vi "Decay Fitter.vi"() -> ()   [LabVIEW 2014]
uses:
  <vilib>/Utility/file.llb/Read From Spreadsheet File (DBL).vi
panel:
  out "time constant":dbl=122.42486013356687
  in  "file path (dialog if empty)":path=path "C:/Users/zchmlk/Desktop/week8-master/Decay2.txt"
  out "Decay Rate Fit":cluster{"all rows":dbl[], "all rows":dbl[]}[](graph)=[{"all rows"=[0.0, 1.0, 2.0, 3.0, 4.0, 5.0, 6.0, 7.0, 8.0, 9.0, 10.0, 11.0, 12.0, 13.0, 14.0, 15.0, 16.0, 17.0, 18.0, 19.0, 20.0, 21.0, 22.0, 23.0, 24.0, 25.0, 26.0, 27.0, 28.0, 29.0, 30.0, 31.0, 32.0, 33.0, 34.0, 35.0, 36.0, 37.0, 38.0, 39.0, 40.0, 41.0, 42.0, 43.0, 44.0, 45.0, 46.0, 47.0, 48.0, 49.0, 50.0, 51.0, 52.0, 53.0, 54.0, 55.0, 56.0, 57.0, 58.0, 59.0, 60.0, 61.0, 62.0, 63.0, 64.0, 65.0, 66.0, 67.0, 68.0, 69.0, 70.0, 71.0, 72.0, 73.0, 74.0, 75.0, 76.0, 77.0, 78.0, 79.0, 80.0, 81.0, 82.0, 83.0, 84.0, 85.0, 86.0, 87.0, 88.0, 89.0, 90.0, 91.0, 92.0, 93.0, 94.0, 95.0, 96.0, 97.0, 98.0, 99.0, 100.0, 101.0, 102.0, 103.0, 104.0, 105.0, 106.0, 107.0, 108.0, 109.0, 110.0, 111.0, 112.0, 113.0, 114.0, 115.0, 116.0, 117.0, 118.0, 119.0, 120.0, 121.0, 122.0, 123.0, 124.0, 125.0, 126.0, 127.0, 128.0, 129.0, 130.0, 131.0, 132.0, 133.0, 134.0, 135.0, 136.0, 137.0, 138.0, 139.0, 140.0, 141.0, 142.0, 143.0, 144.0, 145.0, 146.0, 147.0, 148.0, 149.0, 150.0, 151.0, 152.0, 153.0, 154.0, 155.0, 156.0, 157.0, 158.0, 159.0, 160.0, 161.0, 162.0, 163.0, 164.0, 165.0, 166.0, 167.0, 168.0, 169.0, 170.0, 171.0, 172.0, 173.0, 174.0, 175.0, 176.0, 177.0, 178.0, 179.0, 180.0, 181.0, 182.0, 183.0, 184.0, 185.0, 186.0, 187.0, 188.0, 189.0, 190.0, 191.0, 192.0, 193.0, 194.0, 195.0, 196.0, 197.0, 198.0, 199.0, 200.0, 201.0, 202.0, 203.0, 204.0, 205.0, 206.0, 207.0, 208.0, 209.0, 210.0, 211.0, 212.0, 213.0, 214.0, 215.0, 216.0, 217.0, 218.0, 219.0, 220.0, 221.0, 222.0, 223.0, 224.0, 225.0, 226.0, 227.0, 228.0, 229.0, 230.0, 231.0, 232.0, 233.0, 234.0, 235.0, 236.0, 237.0, 238.0, 239.0, 240.0, 241.0, 242.0, 243.0, 244.0, 245.0, 246.0, 247.0, 248.0, 249.0, 250.0, 251.0, 252.0, 253.0, 254.0, 255.0, 256.0, 257.0, 258.0, 259.0, 260.0, 261.0, 262.0, 263.0, 264.0, 265.0, 266.0, 267.0, 268.0, 269.0, 270.0, 271.0, 272.0, 273.0, 274.0, 275.0, 276.0, 277.0, 278.0, 279.0, 280.0, 281.0, 282.0, 283.0, 284.0, 285.0, 286.0, 287.0, 288.0, 289.0, 290.0, 291.0, 292.0, 293.0, 294.0, 295.0, 296.0, 297.0, 298.0, 299.0, 300.0], "all rows"=[0.0, 74.0, 69.0, 76.0, 68.0, 73.0, 72.0, 70.0, 67.0, 74.0, 72.0, 58.0, 65.0, 66.0, 75.0, 62.0, 69.0, 74.0, 60.0, 56.0, 69.0, 53.0, 65.0, 78.0, 45.0, 64.0, 59.0, 65.0, 63.0, 69.0, 59.0, 56.0, 46.0, 53.0, 49.0, 52.0, 53.0, 47.0, 69.0, 57.0, 53.0, 58.0, 56.0, 56.0, 52.0, 49.0, 51.0, 48.0, 45.0, 50.0, 38.0, 67.0, 58.0, 50.0, 49.0, 46.0, 51.0, 46.0, 50.0, 53.0, 57.0, 43.0, 38.0, 39.0, 48.0, 38.0, 45.0, 43.0, 47.0, 46.0, 34.0, 49.0, 43.0, 45.0, 31.0, 45.0, 24.0, 29.0, 40.0, 40.0, 43.0, 44.0, 36.0, 41.0, 29.0, 42.0, 30.0, 44.0, 50.0, 34.0, 37.0, 30.0, 36.0, 36.0, 34.0, 26.0, 38.0, 31.0, 38.0, 31.0, 42.0, 34.0, 37.0, 31.0, 37.0, 29.0, 40.0, 43.0, 26.0, 28.0, 35.0, 32.0, 35.0, 30.0, 27.0, 26.0, 27.0, 32.0, 33.0, 33.0, 27.0, 33.0, 22.0, 31.0, 34.0, 33.0, 34.0, 23.0, 29.0, 24.0, 26.0, 21.0, 28.0, 33.0, 20.0, 26.0, 19.0, 25.0, 21.0, 30.0, 24.0, 25.0, 23.0, 31.0, 17.0, 31.0, 24.0, 27.0, 20.0, 19.0, 20.0, 23.0, 28.0, 22.0, 25.0, 14.0, 21.0, 30.0, 23.0, 27.0, 22.0, 27.0, 26.0, 22.0, 15.0, 19.0, 19.0, 20.0, 26.0, 19.0, 18.0, 17.0, 18.0, 16.0, 17.0, 22.0, 14.0, 19.0, 17.0, 27.0, 20.0, 16.0, 16.0, 20.0, 22.0, 14.0, 14.0, 26.0, 15.0, 15.0, 17.0, 12.0, 16.0, 19.0, 19.0, 18.0, 11.0, 18.0, 21.0, 14.0, 17.0, 19.0, 10.0, 15.0, 22.0, 26.0, 18.0, 14.0, 23.0, 17.0, 20.0, 16.0, 15.0, 12.0, 9.0, 15.0, 16.0, 14.0, 13.0, 13.0, 21.0, 10.0, 21.0, 15.0, 20.0, 16.0, 12.0, 15.0, 18.0, 18.0, 19.0, 19.0, 20.0, 13.0, 12.0, 9.0, 9.0, 12.0, 13.0, 11.0, 16.0, 14.0, 17.0, 19.0, 16.0, 18.0, 23.0, 13.0, 12.0, 15.0, 9.0, 13.0, 9.0, 21.0, 8.0, 7.0, 17.0, 6.0, 11.0, 11.0, 15.0, 9.0, 20.0, 12.0, 16.0, 15.0, 6.0, 13.0, 9.0, 12.0, 11.0, 10.0, 16.0, 15.0, 12.0, 13.0, 11.0, 12.0, 12.0, 11.0, 13.0, 12.0, 13.0, 8.0, 13.0, 8.0, 15.0, 12.0, 14.0, 13.0, 13.0, 17.0, 12.0, 18.0, 12.0, 8.0, 10.0, 15.0, 13.0, 13.0, 0.0]}, {"all rows"=[0.0, 1.0, 2.0, 3.0, 4.0, 5.0, 6.0, 7.0, 8.0, 9.0, 10.0, 11.0, 12.0, 13.0, 14.0, 15.0, 16.0, 17.0, 18.0, 19.0, 20.0, 21.0, 22.0, 23.0, 24.0, 25.0, 26.0, 27.0, 28.0, 29.0, 30.0, 31.0, 32.0, 33.0, 34.0, 35.0, 36.0, 37.0, 38.0, 39.0, 40.0, 41.0, 42.0, 43.0, 44.0, 45.0, 46.0, 47.0, 48.0, 49.0, 50.0, 51.0, 52.0, 53.0, 54.0, 55.0, 56.0, 57.0, 58.0, 59.0, 60.0, 61.0, 62.0, 63.0, 64.0, 65.0, 66.0, 67.0, 68.0, 69.0, 70.0, 71.0, 72.0, 73.0, 74.0, 75.0, 76.0, 77.0, 78.0, 79.0, 80.0, 81.0, 82.0, 83.0, 84.0, 85.0, 86.0, 87.0, 88.0, 89.0, 90.0, 91.0, 92.0, 93.0, 94.0, 95.0, 96.0, 97.0, 98.0, 99.0, 100.0, 101.0, 102.0, 103.0, 104.0, 105.0, 106.0, 107.0, 108.0, 109.0, 110.0, 111.0, 112.0, 113.0, 114.0, 115.0, 116.0, 117.0, 118.0, 119.0, 120.0, 121.0, 122.0, 123.0, 124.0, 125.0, 126.0, 127.0, 128.0, 129.0, 130.0, 131.0, 132.0, 133.0, 134.0, 135.0, 136.0, 137.0, 138.0, 139.0, 140.0, 141.0, 142.0, 143.0, 144.0, 145.0, 146.0, 147.0, 148.0, 149.0, 150.0, 151.0, 152.0, 153.0, 154.0, 155.0, 156.0, 157.0, 158.0, 159.0, 160.0, 161.0, 162.0, 163.0, 164.0, 165.0, 166.0, 167.0, 168.0, 169.0, 170.0, 171.0, 172.0, 173.0, 174.0, 175.0, 176.0, 177.0, 178.0, 179.0, 180.0, 181.0, 182.0, 183.0, 184.0, 185.0, 186.0, 187.0, 188.0, 189.0, 190.0, 191.0, 192.0, 193.0, 194.0, 195.0, 196.0, 197.0, 198.0, 199.0, 200.0, 201.0, 202.0, 203.0, 204.0, 205.0, 206.0, 207.0, 208.0, 209.0, 210.0, 211.0, 212.0, 213.0, 214.0, 215.0, 216.0, 217.0, 218.0, 219.0, 220.0, 221.0, 222.0, 223.0, 224.0, 225.0, 226.0, 227.0, 228.0, 229.0, 230.0, 231.0, 232.0, 233.0, 234.0, 235.0, 236.0, 237.0, 238.0, 239.0, 240.0, 241.0, 242.0, 243.0, 244.0, 245.0, 246.0, 247.0, 248.0, 249.0, 250.0, 251.0, 252.0, 253.0, 254.0, 255.0, 256.0, 257.0, 258.0, 259.0, 260.0, 261.0, 262.0, 263.0, 264.0, 265.0, 266.0, 267.0, 268.0, 269.0, 270.0, 271.0, 272.0, 273.0, 274.0, 275.0, 276.0, 277.0, 278.0, 279.0, 280.0, 281.0, 282.0, 283.0, 284.0, 285.0, 286.0, 287.0, 288.0, 289.0, 290.0, 291.0, 292.0, 293.0, 294.0, 295.0, 296.0, 297.0, 298.0, 299.0, 300.0], "all rows"=[71.29414997998312, 70.75100442824453, 70.21227736877454, 69.6779328571125, 69.14793524120608, 68.6222491590327, 68.10083953623999, 67.58367158380564, 67.07071079571627, 66.56192294666508, 66.0572740897684, 65.5567305543006, 65.06025894344765, 64.56782613207878, 64.07939926453633, 63.594945752443664, 63.11443327253072, 62.63782976447747, 62.165103428774785, 61.69622272460269, 61.23115636772599, 60.769873328406945, 60.312342829334895, 59.85853434357277, 59.40841759252035, 58.96196254389396, 58.51913940972277, 58.07991864436127, 57.644270942517906, 57.212167237299894, 56.78357869827377, 56.358476729541806, 55.93683296783411, 55.51861928061608, 55.10380776421155, 54.69237074194088, 54.284280762274335, 53.87951059700062, 53.478033239410024, 53.07982190249264, 52.68485001715101, 52.293091230427436, 51.90451940374571, 51.519108611167084, 51.136833137660474, 50.75766747738673, 50.38158633199686, 50.008564608944056, 49.63857741980958, 49.27160007864207, 48.90760810031057, 48.54657719887079, 48.188483285944756, 47.83330246911355, 47.48101105032326, 47.13158552430379, 46.7850025770005, 46.441239084018804, 46.10027210908112, 45.76207890249667, 45.42663689964354, 45.09392371946312, 44.763917162966905, 44.436595211755204, 44.11193602654821, 43.78991794572876, 43.470519483897064, 43.15371933043723, 42.83949634809527, 42.52782957156896, 42.21869820610891, 41.912081626131126, 41.60795937384087, 41.30631115786768, 41.00711685191153, 40.71035649339994, 40.41601028215608, 40.1240585790777, 39.83448190482672, 39.54726093852962, 39.2623765164883, 38.97980963090147, 38.69954142859635, 38.42155320977092, 38.1458264267461, 37.87234268272829, 37.60108373058196, 37.3320314716121, 37.065167954356696, 36.80047537338898, 36.53793606812944, 36.277532521667496, 36.019247359592704, 35.76306334883559, 35.50896339651778, 35.25693054881157, 35.00694798980875, 34.75899904039862, 34.513067157155135, 34.26913593123314, 34.0271890872735, 33.78721048231726, 33.549184104728496, 33.31309407312607, 33.078924635323936, 32.846660167280206, 32.61628517205466, 32.38778427877476, 32.16114224161012, 31.936343938755286, 31.713374371420755, 31.49221866283228, 31.272862057238253, 31.05528991892521, 30.83948773124128, 30.62544109562765, 30.413135730657874, 30.202557471084987, 29.993692266896392, 29.786526182376427, 29.581045395176563, 29.377236195393152, 29.1750849846527, 28.974578275204564, 28.775702689021013, 28.578444956904683, 28.38279191760317, 28.18873051693096, 27.996247806898428, 27.80533094484788, 27.615967192596763, 27.428143915587682, 27.24184858204545, 27.057068762140958, 26.873792127161806, 26.692006448689767, 26.511699597784855, 26.33285954417608, 26.155474355458782, 25.979532196298496, 25.805021327641246, 25.631930105930348, 25.460246982329515, 25.28996050195231, 25.121059303097876, 24.95353211649284, 24.78736776453945, 24.622555160569775, 24.459083308105985, 24.296941300126665, 24.136118318339093, 23.97660363245742, 23.818386599486715, 23.661456663012903, 23.505803352498383, 23.351416282583436, 23.198285152393325, 23.046399744850966, 22.89574992599527, 22.74632564430498, 22.59811693002803, 22.45111389451633, 22.305306729566016, 22.160685706763008, 22.01724117683394, 21.87496356900235, 21.733843390350074, 21.59387122518391, 21.455037734407387, 21.317333654897613, 21.180749798887266, 21.04527705335158, 20.910906379400277, 20.777628811674518, 20.645435457748707, 20.514317497537185, 20.384266182705737, 20.255272836087904, 20.12732885110602, 20.000425691196995, 19.874554889242702, 19.749708047005104, 19.625876834565858, 19.503052989770552, 19.38122831767747, 19.260394690010777, 19.140544044618217, 19.021668384933193, 18.903759779441213, 18.786810361150714, 18.67081232706815, 18.55575793767738, 18.441639516423265, 18.328449449199482, 18.216180183840528, 18.104824229617794, 17.994374156739795, 17.88482259585645, 17.776162237567373, 17.66838583193421, 17.56148618799688, 17.45545617329382, 17.350288713386075, 17.245976791385292, 17.142513447485555, 17.039891778499, 16.93810493739524, 16.83714613284453, 16.737008628764613, 16.637685743871323, 16.53917085123276, 16.441457377827177, 16.344538804104374, 16.248408663550737, 16.153060542257794, 16.058488078494236, 15.964684962281488, 15.87164493497268, 15.779361788835079, 15.68782936663589, 15.597041561231443, 15.506992315159717, 15.417675620236189, 15.329085517152937, 15.241216095081054, 15.154061491276266, 15.067615890687746, 14.981873525570146, 14.896828675098764, 14.812475664987833, 14.728808867111937, 14.6458226991305, 14.563511624115309, 14.4818701501811, 14.400892830119133, 14.320574261033732, 14.240909083981819, 14.161891983615343, 14.083517687826642, 14.005780967396692, 13.928676635646173, 13.852199548089457, 13.776344602091324, 13.701106736526521, 13.626480931442078, 13.552462207722385, 13.479045626756948, 13.406226290110913, 13.333999339198213, 13.26235995495742, 13.191303357530181, 13.120824805942332, 13.050919597787559, 12.98158306891365, 12.9128105931113, 12.844597581805447, 12.776939483749103, 12.70983178471971, 12.64327000721794, 12.577249710168942, 12.511766488626035, 12.446815973476815, 12.382393831151617, 12.318495763334404, 12.255117506675958, 12.192254832509438, 12.12990354656823, 12.0680594887061, 12.006718532619633, 11.945876585572915, 11.885529588124463, 11.825673513856376, 11.766304369105685, 11.707418192697887, 11.649011055682667, 11.591079061071738, 11.533618343578837, 11.47662506936183, 11.42009543576691, 11.364025671074877, 11.308412034249491, 11.253250814687867, 11.198538331972895, 11.14427093562768, 11.09044500487198, 11.037056948380611, 10.984103204043855, 10.931580238729769, 10.87948454804846, 10.827812656118276, 10.77656111533387, 10.725726506136187, 10.675305436784317, 10.625294543129167, 10.575690488389027, 10.526489962926924, 10.477689684029796, 10.429286395689477, 10.381276868385445, 10.333657898869344, 10.286426309951267]}]
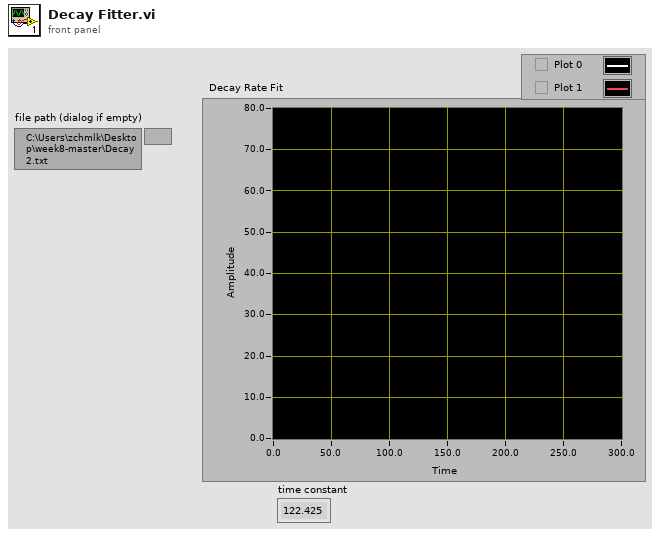
[diagram p1: front panel]
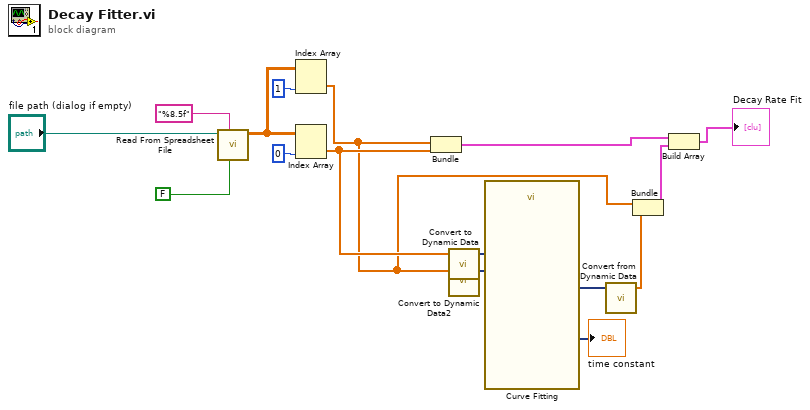
[diagram p0: block diagram]
diagram:
  n1 = call-poly <vilib>:"Read From Spreadsheet File.vi"("transpose (no:F)"=FALSE, "format (%.3f)"="%8.5f", "file path (dialog if empty)"="file path (dialog if empty)") -> ("all rows"=w14:dbl[][])  [unwired: 4 in, 4 out]
  n2 = Index Array(array=w14, index (col)=1) -> (element=w4:dbl[])  [unwired: 1 in]
  n3 = Index Array(array=w14, index (col)=0) -> (element=w8:dbl[])  [unwired: 1 in]
  n4 = Bundle("all rows"=w4, "all rows"=w8) -> (w7:cluster{"all rows":dbl[], "all rows":dbl[]})  [unwired: 1 in]
  n5 = call "Convert to Dynamic Data"("Array"=w8) -> ("Dynamic Data Type"=w10:dynamicdata)  [unwired: 3 in]
  n6 = call "Convert to Dynamic Data2"("Array"=w4) -> ("Dynamic Data Type"=w9:dynamicdata)  [unwired: 3 in]
  n7 = call "Curve Fitting"("Locations"=w9, "Signals"=w10) -> ("best fit"=w5:dynamicdata, "non-linear coefficients"=→"time constant":dynamicdata)  [unwired: 5 in, 3 out]
  n8 = call "Convert from Dynamic Data"("Dynamic Data Type"=w5) -> ("Array"=w3:dbl[])  [unwired: 3 in]
  n9 = Bundle("all rows"=w4, "Array"=w3) -> (w2:cluster{"all rows":dbl[], "Array":dbl[]})  [unwired: 1 in]
  n10 = Build Array(w7, w2) -> (→"Decay Rate Fit":cluster{"all rows":dbl[], "Array":dbl[]}[])
